vi "UART_SDI_12_wave_collection.vi"() -> (2 "soil moisture saved":bool=TRUE)   [LabVIEW 2019]
uses:
  <vilib>/myRIO/Instrument Drivers/Onboard IO/UART/typedef/VISA Configuration.ctl
  <vilib>/myRIO/Instrument Drivers/Onboard IO/DIO/typedefs/DIO Reference.ctl
  <vilib>/myRIO/Common/Instrument Driver Framework/Utilities/typedefs/myRIO Generic Hardware Reference.ctl
  <vilib>/myRIO/Common/Instrument Driver Framework/Utilities/typedefs/Hardware Version Enum.ctl
  <vilib>/myRIO/Common/Instrument Driver Framework/Utilities/typedefs/myRIO v1.0 Reference.ctl
  <vilib>/myRIO/Common/Instrument Driver Framework/Utilities/typedefs/Generic FPGA Reference.ctl
  <vilib>/myRIO/Common/Instrument Driver Framework/myRIO v1.0/DIO/typedefs/DIO Channels List.ctl
  <vilib>/myRIO/Common/Instrument Driver Framework/myRIO v1.0/DIO/typedefs/DIO Channels Enum.ctl
  <vilib>/userdefined/High Color/nirio_resource_hc.ctl
  <vilib>/myRIO/Common/Instrument Driver Framework/Utilities/vis/Is FPGA Ref Available.vi
  <vilib>/myRIO/Common/Instrument Driver Framework/myRIO v1.0/DIO/vis/myRIO v1.1 Open DIO.vi
  <vilib>/myRIO/Instrument Drivers/Onboard IO/DIO/vis/Write.vi
  <vilib>/myRIO/Common/Instrument Driver Framework/Utilities/vis/Validate Channels.vi
  <vilib>/myRIO/Common/Instrument Driver Framework/myRIO v1.0/DIO/vis/myRIO v1.0 Reserve DIO.vi
  <vilib>/myRIO/Common/Instrument Driver Framework/myRIO v1.0/Resource Manager/vis/myRIO v1.0 Reserve Channel List.vi
  <vilib>/myRIO/Common/Instrument Driver Framework/myRIO v1.0/DIO/vis/myRIO v1.0 Build MUX Configuration DIO.vi
  <vilib>/myRIO/Common/Instrument Driver Framework/myRIO v1.0/Resource Manager/vis/myRIO v1.0 Reserve Channel.vi
  <vilib>/myRIO/Common/Instrument Driver Framework/myRIO v1.0/Resource Manager/vis/myRIO v1.0 Unreserve Channel.vi
  <vilib>/myRIO/Common/Instrument Driver Framework/myRIO v1.0/Resource Manager/vis/myRIO v1.0 Create Configuration List.vi
  <vilib>/myRIO/Common/Instrument Driver Framework/myRIO v1.0/Resource Manager/vis/myRIO v1.0 Build Mutex Name.vi
  <vilib>/Instr/_visa.llb/VISA Configure Serial Port (Instr).vi
  <vilib>/Utility/VariantDataType/GetNumericInfo.vi
  <vilib>/Utility/error.llb/Error Cluster From Error Code.vi
  <vilib>/myRIO/Common/Instrument Driver Framework/myRIO v1.0/myRIO v1.1 Open.vi
  <vilib>/myRIO/Common/Instrument Driver Framework/Utilities/vis/IO Manager.vi
  <vilib>/myRIO/Common/Instrument Driver Framework/Utilities/vis/Configuration Manager.vi
  <vilib>/myRIO/Common/Instrument Driver Framework/myRIO v1.0/Resource Manager/vis/myRIO v1.0 Configure IO.vi
  <vilib>/myRIO/Common/Instrument Driver Framework/myRIO v1.0/myRIO v1.0 Close.vi
  <vilib>/myRIO/Common/Instrument Driver Framework/myRIO v1.0/DIO/vis/myRIO v1.0 Write DIO.vi
  <vilib>/myRIO/Express VI/Onboard IO/UART/UART Express VI.xnode
  <vilib>/myRIO/Express VI/Onboard Devices/LED/LED Express VI.xnode
  <vilib>/myRIO/Instrument Drivers/Onboard IO/DIO/vis/myRIO DIO Open.xnode
  <vilib>/myRIO/Instrument Drivers/Onboard IO/UART/UART.lvlib
  <vilib>/myRIO/Instrument Drivers/Onboard IO/DIO/DIO.lvlib
panel:
  out "3D1?":bool
  out "Number of 3D0":i32
  out "result string":string
  out "number of replacements":i32
  out "offset past replacement":i32
  out "UART_count":i64
  out "moisture_count":i64
  out "number of iterations":i32
  out "Response from acclima sensor":string
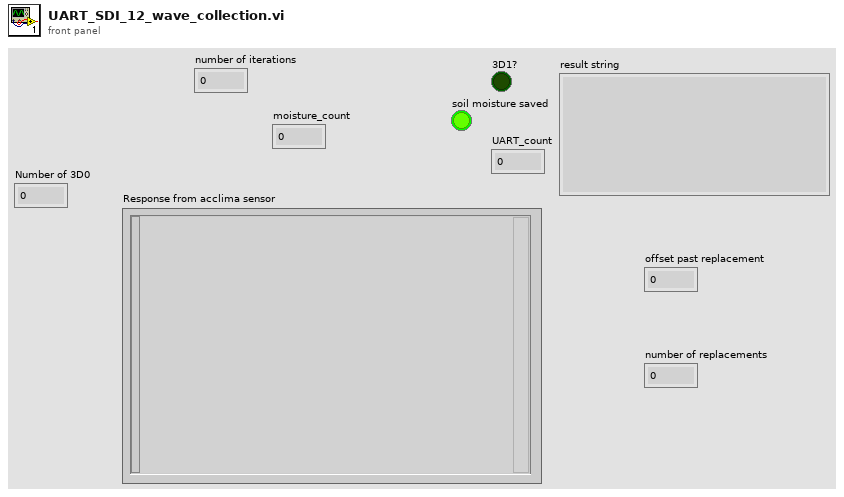
[diagram p1: front panel]
types:
  T1 = enum16{"open", "replace", "create", "open or create", "replace or create", "replace or create with confirmation"}
  T2 = typedef "UART.lvlib/VISA Configuration.ctl" = cluster{"baud rate (9600)":u32, "data bits (8)":u16, "parity (0:none)":enum16{"None", "Odd", "Even", "Mark", "Space"}, "stop bits (10: 1 bit)":u16, "flow control (0:none)":u16, "termination char\n(0xA = '\\n' = LF) ":u8, "Enable Termination\nChar (T)":bool, "timeout (10sec)":u32}
  T3 = typedef "DIO.lvlib/DIO Reference.ctl" = cluster{"myRIO Reference":T4, "DIO Channels List":T8}
  T4 = typedef "myRIO Generic Hardware Reference.ctl" = cluster{"myRIO Model":T5, "myRIO Hardware Reference":T6}
  T5 = typedef "Hardware Version Enum.ctl" = enum16{"Unknown", "myRIO-1900", "myRIO-1950", "roboRIO", "NI ELVIS RIO CM", "ELVIS III"}
  T6 = typedef "myRIO v1.0 Reference.ctl" = cluster{"Generic FPGA Reference":T7, "Allow multiple opens":bool}
  T7 = typedef "Generic FPGA Reference.ctl" = refnum<k20>
  T8 = typedef "DIO Channels List.ctl" = T9[]
  T9 = typedef "DIO Channels Enum.ctl" = enum16{"Not Connected", "C/DIO0", "C/DIO1", "C/DIO2", "C/DIO3", "C/DIO4", "C/DIO5", "C/DIO6", "C/DIO7", "A/DIO0", "A/DIO1", "A/DIO2", "A/DIO3", "A/DIO4", "A/DIO5", "A/DIO6", "A/DIO7", "A/DIO8", "A/DIO9", "A/DIO10", "A/DIO11", "A/DIO12", "A/DIO13", "A/DIO14", "A/DIO15", "A/DIO16", "A/DIO17", "A/DIO18", "A/DIO19", "B/DIO0", "B/DIO1", "B/DIO2", "B/DIO3", "B/DIO4", "B/DIO5", "B/DIO6", "B/DIO7", "B/DIO8", "B/DIO9", "B/DIO10", "B/DIO11", "B/DIO12", "B/DIO13", "B/DIO14", "B/DIO15", "B/DIO16", "B/DIO17", "B/DIO18", "B/DIO19", "LED0", "LED1", "LED2", "LED3", "Button0", "DIO/DIO0", "DIO/DIO1", "DIO/DIO2", "DIO/DIO3", "DIO/DIO4", "DIO/DIO5", "DIO/DIO6", "DIO/DIO7", "DIO/DIO8", "DIO/DIO9", "SPI/CS0", "SPI/CS1", "SPI/CS2", "SPI/CS3", "LED RADIO (Green)", "LED RADIO (Red)", "LED COMM (Green)", "LED COMM (Red)", "LED MODE (Green)", "LED MODE (Red)"}
  T10 = typedef "nirio_resource_hc.ctl" = tag
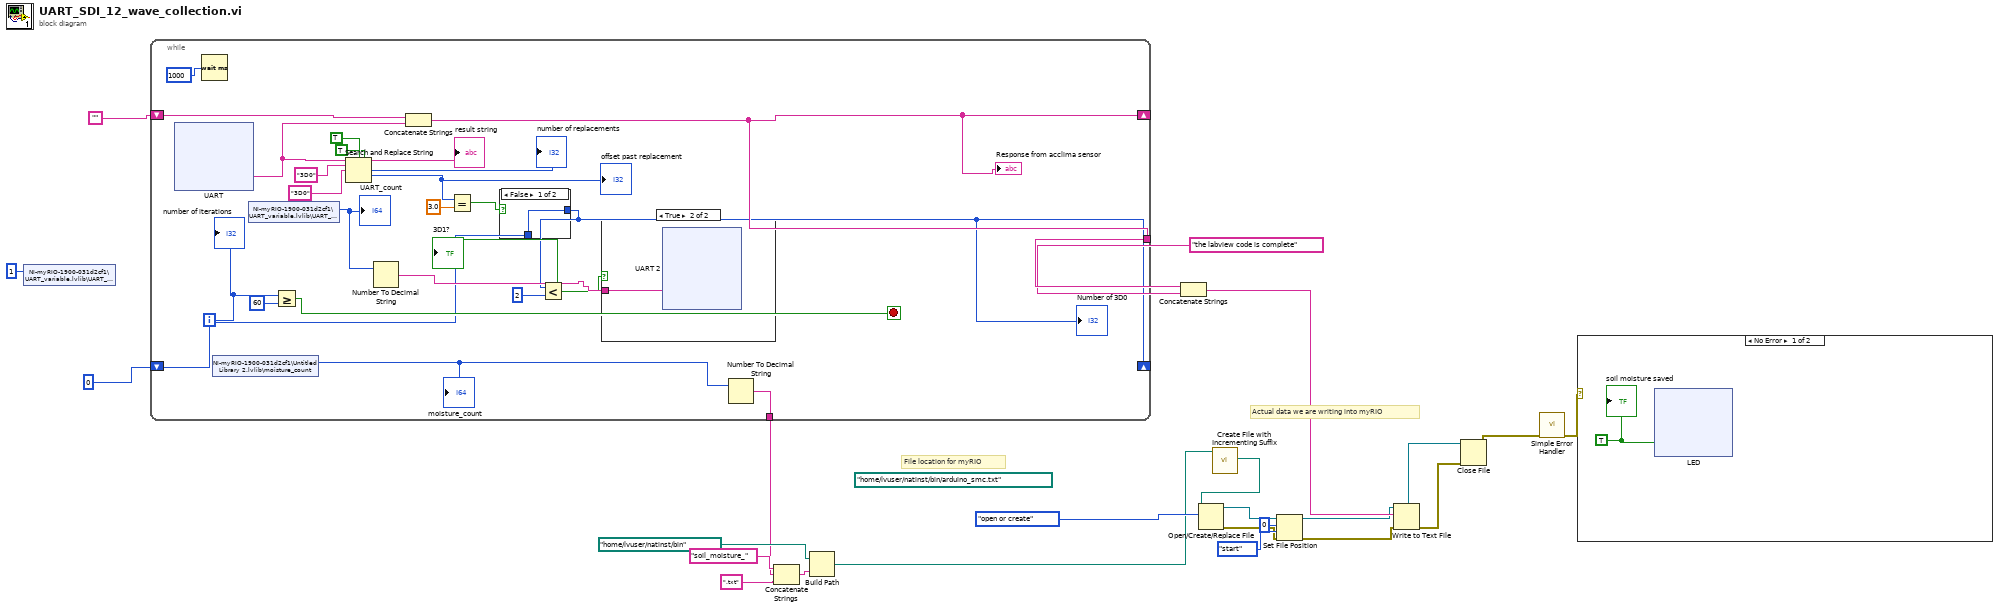
[diagram p0: block diagram]
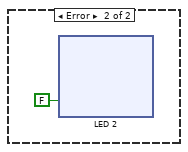
[diagram p2: hidden frame]
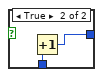
[diagram p3: hidden frame]
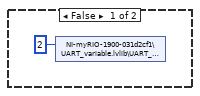
[diagram p4: hidden frame]
diagram:
  (unwired) path "/home/lvuser/natinst/bin/arduino_smc.txt" ("file path (use dialog)")
  # "Actual data we are writing into myRIO"
  # "File location for myRIO"
  n1 = shared-variable "NI-myRIO-1900-031d2cf1\\UART_variable.lvlib\\UART_count"(i64 1 ("UART_count")) -> ()  [unwired: 1 in, 1 out]
  n2 = while {
    tunnel: [w31] -> w20
    tunnel: [w44] -> w5
    shift-right: [w31] -> _
    shift-left: "" -> [w43]
    shift-right: [w26] -> _
    shift-left: 0 -> [w25]
    i -> [w42]
    stop <- w45 stop-if-true
    n3 = xnode "UART"() -> ("Characters Read"=w35:string)  [unwired: 1 in, 1 out]
    n4 = Wait (ms)(milliseconds to wait=u32 1000) -> ()  [unwired: 1 out]
    n5 = shared-variable "NI-myRIO-1900-031d2cf1\\Untitled Library 2.lvlib\\moisture_count"() -> (w41:i64)  [unwired: 1 in, 1 out]
    "moisture_count" <- w41
    n6 = shared-variable "NI-myRIO-1900-031d2cf1\\UART_variable.lvlib\\UART_count"() -> (w30:i64)  [unwired: 1 in, 1 out]
    "UART_count" <- w30
    n7 = Greater Or Equal?(x=w42, y=60) -> (x >= y?=w45:bool)
    n8 = Search and Replace String(case sensitive?=TRUE ("ignore case? (F)"), multiline?=TRUE ("multiline? (F)"), input string=w35, search string="3D0", replace string="3D0" ("replace string (\"\")")) -> (result string=→"result string":string, number of replacements=→"number of replacements":i32, offset past replacement=w32:i32)  [unwired: 3 in, 1 out]
    "offset past replacement" <- w32
    n9 = Number To Decimal String(number=w30) -> (decimal integer string=w29:string)  [unwired: 1 in]
    n10 = Concatenate Strings(w43, w35) -> (w31:string)
    "Response from acclima sensor" <- w31
    n11 = Equal?(x=w32, y=3.0) -> (x = y?=w27:bool)
    n12 = case shown="False" w27 {
      tunnel: [w49 w50] -> w26
      tunnel: w25 -> [w49 w51]
      frame False {
      }
      frame True {
        n13 = Increment(x=w51) -> (x+1=w50:i32)
      }
    }
    "Number of 3D0" <- w26
    n14 = Less?(x=w26, y=2) -> (x < y?=w28:bool)
    "3D1?" <- w28
    n15 = case shown="True" w28 {
      tunnel: w29 -> [_ w53]
      frame False {
        n16 = shared-variable "NI-myRIO-1900-031d2cf1\\UART_variable.lvlib\\UART_count"(i64 2 ("UART_count")) -> ()  [unwired: 1 in, 1 out]
      }
      frame True {
        n17 = xnode "UART 2"("Characters to Write"=w53) -> ()  [unwired: 1 in, 2 out]
      }
    }
    n18 = Number To Decimal String(number=w41) -> (decimal integer string=w44:string)  [unwired: 1 in]
    "number of iterations" <- w42
  }
  n19 = Concatenate Strings("soil_moisture_" ("string"), w5, ".txt" ("string")) -> (w8:string)
  n20 = Build Path(base path=path "/home/lvuser/natinst/bin", name or relative path=w8) -> (appended path=w4:path)
  n21 = Concatenate Strings(w20, "the labview code is complete") -> (w17:string)
  n22 = call <vilib>:"Create File with Incrementing Suffix.vi"("file path"=w4) -> ("actual path"=w18:path)  [unwired: 8 in, 2 out]
  n23 = Open/Create/Replace File(file path (use dialog)=w18, operation (0:open)=T1."open or create") -> (refnum out=w15:refnum<file>, error out=w11:errorcluster)  [unwired: 4 in, 1 out]
  n24 = Set File Position(offset (in bytes) (0)=i64 0, refnum=w15, from (0:start)=enum16{"start", "end", "current"}."start", error in=w11) -> (refnum out=w14:refnum<file>, error out=w10:errorcluster)
  n25 = Write to Text File(file (use dialog)=w14, text=w17, error in=w10) -> (refnum out=w23:refnum<file>, error out=w22:errorcluster)  [unwired: 1 in, 1 out]
  n26 = Close File(refnum=w23, error in=w22) -> (error out=w21:errorcluster)  [unwired: 1 out]
  n27 = call <vilib>:"Simple Error Handler.vi"("error in (no error)"=w21) -> ("error out"=w16:errorcluster)  [unwired: 4 in, 4 out]
  n28 = case shown="No Error" w16 {
    frame No Error {
      w87 = TRUE ("LED0")
      n29 = xnode "LED"("LED0"=w87) -> ()  [unwired: 1 in, 1 out]
      "soil moisture saved" <- w87
    }
    frame Error {
      n30 = xnode "LED 2"("LED0"=FALSE) -> ()  [unwired: 1 in, 1 out]
    }
  }
